vi "Msg Post Priority Message.vi"   [LabVIEW 2014]
doc: "Post a high priority message to the front of the specified message queue (or event structure). This function does not await a response from the recipient. It is \"fire and forget.\"\n\nThis is part of the Msg suite, intended to make messaging architectures in LabVIEW\nSee the template \"Message Based Application Template.vi\" for normal usage.\n\nCopyright 2005-2016 Jason Sommerville\n\nThis VI may be freely used, modified or distributed under the BSD license."
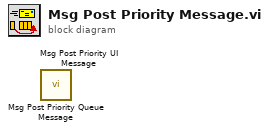
[diagram p0: block diagram]
diagram:
  n1 = call "Msg Post Priority Queue Message.vi"() -> ()  [unwired: 7 in, 3 out]
  n2 = call "Msg Post Priority UI Message.vi"() -> ()  [unwired: 8 in, 2 out]
